vi "Write Block on Wait.vi"(8 "error in (no error)":errorcluster, 10 "Block on Wait?":bool, 11 "WriteCommand in":refnum<class "WriteCommand.lvclass">) -> (0 "error out":errorcluster, 3 "WriteCommand out":refnum<class "WriteCommand.lvclass">)   [LabVIEW 2023, in "HAF.lvlib" / "WriteCommand.lvclass"]
doc: "Sets whether or not the Command should block execution whilst it waits for other Commands to finish. The default is to not block."
uses:
  WriteCommand.lvclass
  WriteCommand.lvclass/WriteCommand.ctl
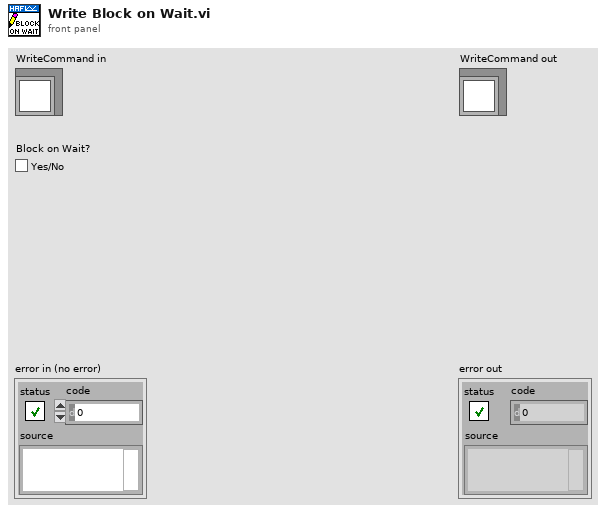
[diagram p1: front panel]
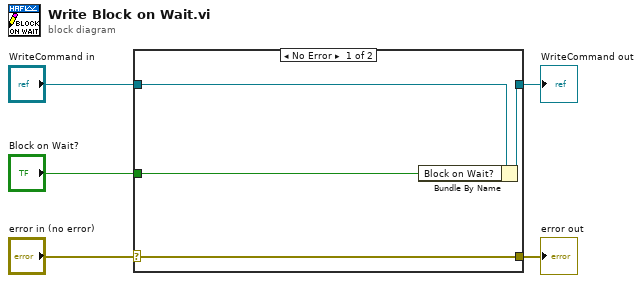
[diagram p0: block diagram]
diagram:
  n1 = case shown="No Error" "error in (no error)" {
    selector: "error in (no error)" -> [w9 w10]
    tunnel: [w9 w10] -> w4
    tunnel: [w7 w11] -> w2
    tunnel: "WriteCommand in" -> [w8 w11]
    tunnel: "Block on Wait?" -> [w6 _]
    frame No Error {
      n2 = Bundle By Name(cluster=w8, "Block on Wait?"=w6) -> (w7:refnum<class "WriteCommand.lvclass">)
    }
    frame Error {
    }
  }
  "error out" <- w4
  "WriteCommand out" <- w2
